vi "subkruispuntbocht.vi"(10 "control 123":i32, 11 "lijn gedetecteerd":bool) -> (9 "einde keuze":bool)   [LabVIEW 2019]
uses:
  <vilib>/myRIO/Common/Instrument Driver Framework/Utilities/typedefs/Analog Scaling Constants.ctl
  <vilib>/myRIO/Common/Instrument Driver Framework/Utilities/typedefs/Analog Scaling Constants List.ctl
  <vilib>/myRIO/Common/Instrument Driver Framework/myRIO v1.0/AO/typedefs/AO Channels Enum.ctl
  <vilib>/myRIO/Common/Instrument Driver Framework/myRIO v1.0/AO/typedefs/AO Channels List.ctl
  <vilib>/myRIO/Common/Instrument Driver Framework/Utilities/typedefs/Generic FPGA Reference.ctl
  <vilib>/myRIO/Common/Instrument Driver Framework/Utilities/typedefs/myRIO v1.0 Reference.ctl
  <vilib>/myRIO/Common/Instrument Driver Framework/Utilities/typedefs/Hardware Version Enum.ctl
  <vilib>/myRIO/Common/Instrument Driver Framework/Utilities/typedefs/myRIO Generic Hardware Reference.ctl
  <vilib>/myRIO/Instrument Drivers/Onboard IO/AO/typedefs/AO Reference.ctl
  <vilib>/myRIO/Instrument Drivers/Onboard IO/AO/AO.lvlib
  <vilib>/myRIO/Instrument Drivers/Onboard IO/AO/vis/Write.vi
  <vilib>/userDefined/High Color/nirio_resource_hc.ctl
  <vilib>/myRIO/Common/Instrument Driver Framework/myRIO v1.0/AO/vis/myRIO v1.1 Open AO.vi
  <vilib>/myRIO/Instrument Drivers/Onboard IO/AO/vis/myRIO AO Open.xnode
  <vilib>/myRIO/Common/Instrument Driver Framework/Utilities/vis/Is FPGA Ref Available.vi
  <vilib>/myRIO/Express VI/Onboard IO/AO/AO Express VI.xnode
  <vilib>/myRIO/Common/Instrument Driver Framework/myRIO v1.0/DIO/typedefs/DIO Channels Enum.ctl
  <vilib>/myRIO/Common/Instrument Driver Framework/myRIO v1.0/DIO/typedefs/DIO Channels List.ctl
  <vilib>/myRIO/Instrument Drivers/Onboard IO/DIO/typedefs/DIO Reference.ctl
  <vilib>/myRIO/Instrument Drivers/Onboard IO/DIO/DIO.lvlib
  <vilib>/myRIO/Instrument Drivers/Onboard IO/DIO/vis/Read.vi
  <vilib>/myRIO/Common/Instrument Driver Framework/myRIO v1.0/DIO/vis/myRIO v1.1 Open DIO.vi
  <vilib>/myRIO/Instrument Drivers/Onboard IO/DIO/vis/myRIO DIO Open.xnode
  <vilib>/myRIO/Express VI/Onboard IO/DI/DI Express VI.xnode
  <vilib>/myRIO/Instrument Drivers/Onboard IO/I2C/typedefs/I2C Transfer Rate.ctl
  <vilib>/myRIO/Instrument Drivers/Onboard IO/I2C/I2C.lvlib
  <vilib>/myRIO/Instrument Drivers/Onboard IO/I2C/typedefs/I2C User Configuration.ctl
  <vilib>/myRIO/Instrument Drivers/Onboard IO/I2C/typedefs/I2C Configuration.ctl
  <vilib>/myRIO/Common/Instrument Driver Framework/myRIO v1.0/I2C/typedefs/I2C Channels Enum.ctl
  <vilib>/myRIO/Instrument Drivers/Onboard IO/I2C/typedefs/I2C Reference.ctl
  <vilib>/myRIO/Instrument Drivers/Onboard IO/I2C/vis/Configure.vi
  <vilib>/myRIO/Instrument Drivers/Onboard IO/I2C/vis/Write.vi
  <vilib>/myRIO/Common/Instrument Driver Framework/myRIO v1.0/I2C/vis/myRIO v1.1 Open I2C.vi
  <vilib>/myRIO/Instrument Drivers/Onboard IO/I2C/vis/myRIO I2C Open.xnode
  <vilib>/myRIO/Express VI/Onboard IO/I2C/I2C Express VI.xnode
  stopkruispunt.vi
panel:
  out "rood  5":u32
  out "rood  4":u32
  out "rood  3":u32
  in  "error in (no error) 4":errorcluster
  out "error out 4":errorcluster
  in  "error in (no error) 3":errorcluster
  out "error out 3":errorcluster
  in  "error in (no error) 2":errorcluster
  out "error out 2":errorcluster
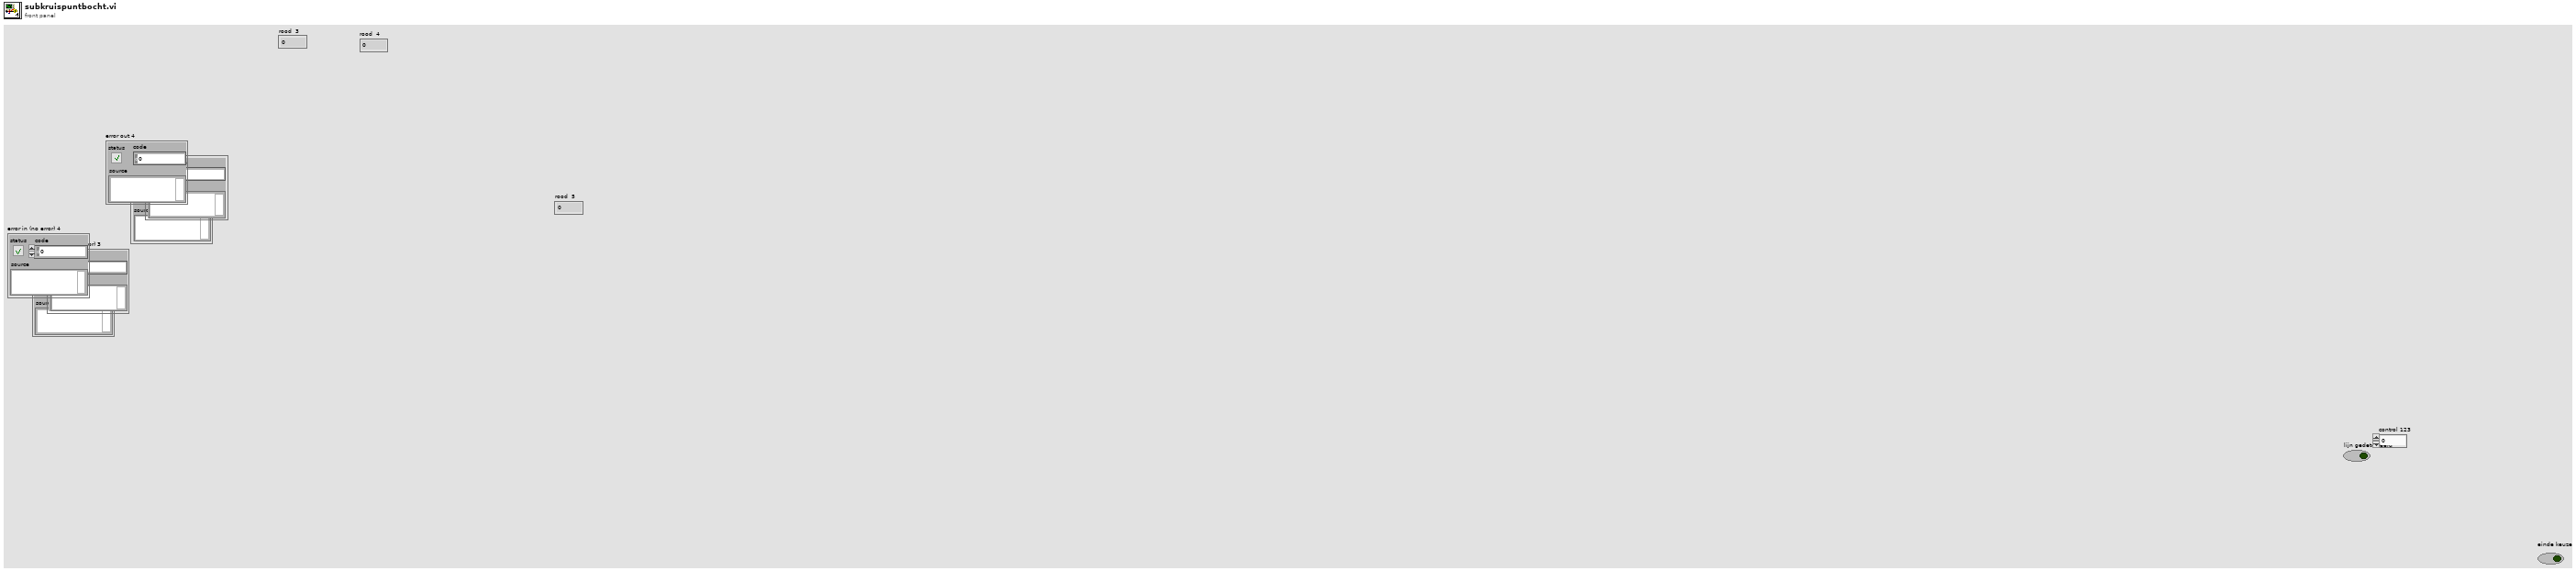
[diagram p1: front panel]
types:
  T1 = typedef "AO.lvlib/AO Reference.ctl" = cluster{"myRIO Reference":T2, "AO Channel List":T6, "AO Scaling Constant List":T8}
  T2 = typedef "myRIO Generic Hardware Reference.ctl" = cluster{"myRIO Model":T3, "myRIO Hardware Reference":T4}
  T3 = typedef "Hardware Version Enum.ctl" = enum16{"Unknown", "myRIO-1900", "myRIO-1950", "roboRIO", "NI ELVIS RIO CM", "ELVIS III"}
  T4 = typedef "myRIO v1.0 Reference.ctl" = cluster{"Generic FPGA Reference":T5, "Allow multiple opens":bool}
  T5 = typedef "Generic FPGA Reference.ctl" = refnum<k20>
  T6 = typedef "AO Channels List.ctl" = T7[]
  T7 = typedef "AO Channels Enum.ctl" = enum16{"Not Connected", "AudioOut/Left", "AudioOut/Right", "C/AO0", "C/AO1", "A/AO0", "A/AO1", "B/AO0", "B/AO1"}
  T8 = typedef "Analog Scaling Constants List.ctl" = T9[]
  T9 = typedef "Analog Scaling Constants.ctl" = cluster{"LSB Weight (Volts)":dbl, "Offset (Volts)":dbl, "Signed?":bool}
  T10 = typedef "nirio_resource_hc.ctl" = tag
  T11 = typedef "I2C.lvlib/I2C Reference.ctl" = cluster{"myRIO Reference":T2, "I2C Channels Enum":T12, "I2C Configuration":T13}
  T12 = typedef "I2C Channels Enum.ctl" = enum16{"Not Connected", "A/I2C", "B/I2C", "I2C/I2C"}
  T13 = typedef "I2C.lvlib/I2C Configuration.ctl" = cluster{"I2C Transfer Rate":T14}
  T14 = typedef "I2C.lvlib/I2C Transfer Rate.ctl" = enum16{"Standard mode (100 kbps)", "Fast mode (400 kbps)"}
  T15 = typedef "I2C.lvlib/I2C User Configuration.ctl" = cluster{"I2C Transfer Rate":T14}
  T16 = typedef "DIO.lvlib/DIO Reference.ctl" = cluster{"myRIO Reference":T2, "DIO Channels List":T17}
  T17 = typedef "DIO Channels List.ctl" = T18[]
  T18 = typedef "DIO Channels Enum.ctl" = enum16{"Not Connected", "C/DIO0", "C/DIO1", "C/DIO2", "C/DIO3", "C/DIO4", "C/DIO5", "C/DIO6", "C/DIO7", "A/DIO0", "A/DIO1", "A/DIO2", "A/DIO3", "A/DIO4", "A/DIO5", "A/DIO6", "A/DIO7", "A/DIO8", "A/DIO9", "A/DIO10", "A/DIO11", "A/DIO12", "A/DIO13", "A/DIO14", "A/DIO15", "A/DIO16", "A/DIO17", "A/DIO18", "A/DIO19", "B/DIO0", "B/DIO1", "B/DIO2", "B/DIO3", "B/DIO4", "B/DIO5", "B/DIO6", "B/DIO7", "B/DIO8", "B/DIO9", "B/DIO10", "B/DIO11", "B/DIO12", "B/DIO13", "B/DIO14", "B/DIO15", "B/DIO16", "B/DIO17", "B/DIO18", "B/DIO19", "LED0", "LED1", "LED2", "LED3", "Button0", "DIO/DIO0", "DIO/DIO1", "DIO/DIO2", "DIO/DIO3", "DIO/DIO4", "DIO/DIO5", "DIO/DIO6", "DIO/DIO7", "DIO/DIO8", "DIO/DIO9", "SPI/CS0", "SPI/CS1", "SPI/CS2", "SPI/CS3", "LED RADIO (Green)", "LED RADIO (Red)", "LED COMM (Green)", "LED COMM (Red)", "LED MODE (Green)", "LED MODE (Red)"}
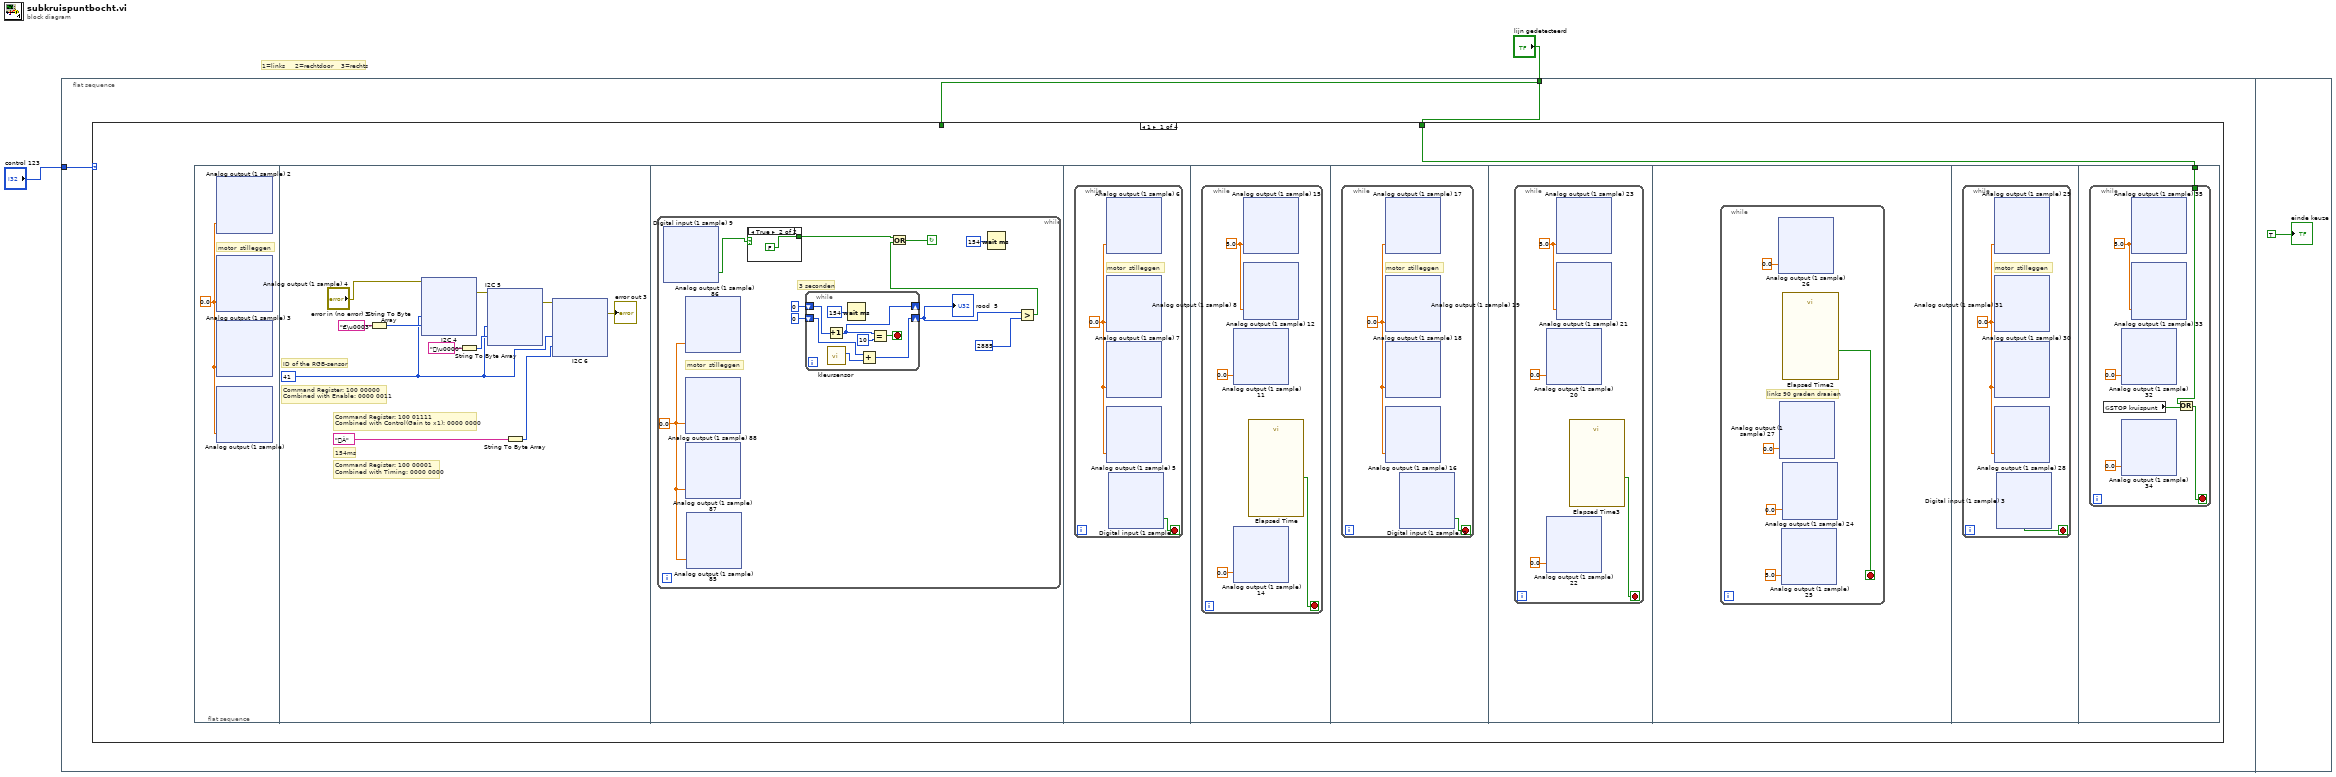
[diagram p0: block diagram]
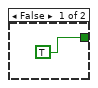
[diagram p2: hidden frame]
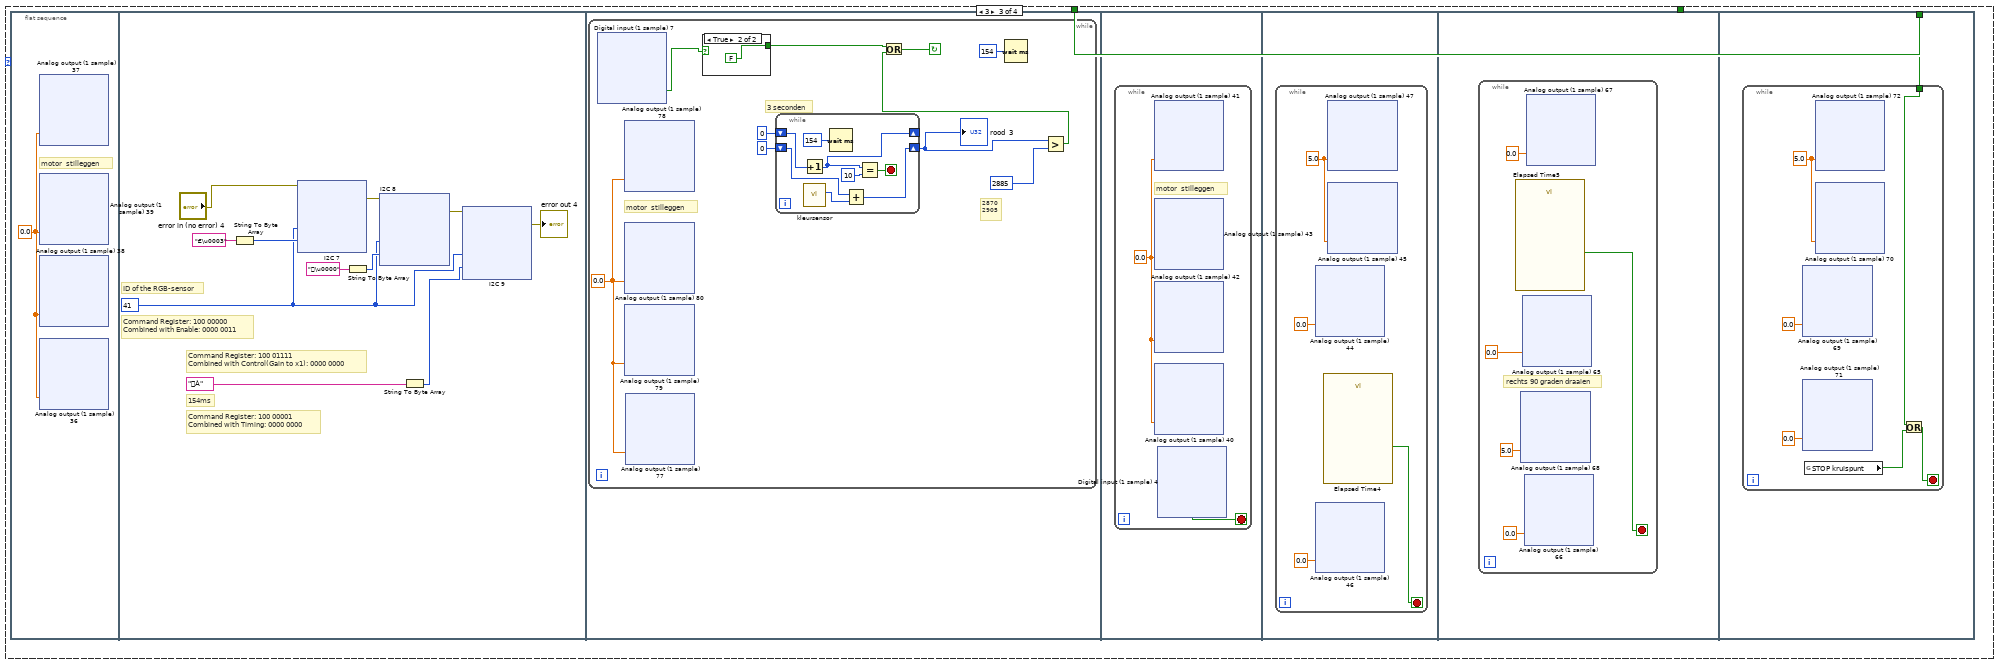
[diagram p4: hidden frame]
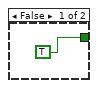
[diagram p5: hidden frame]
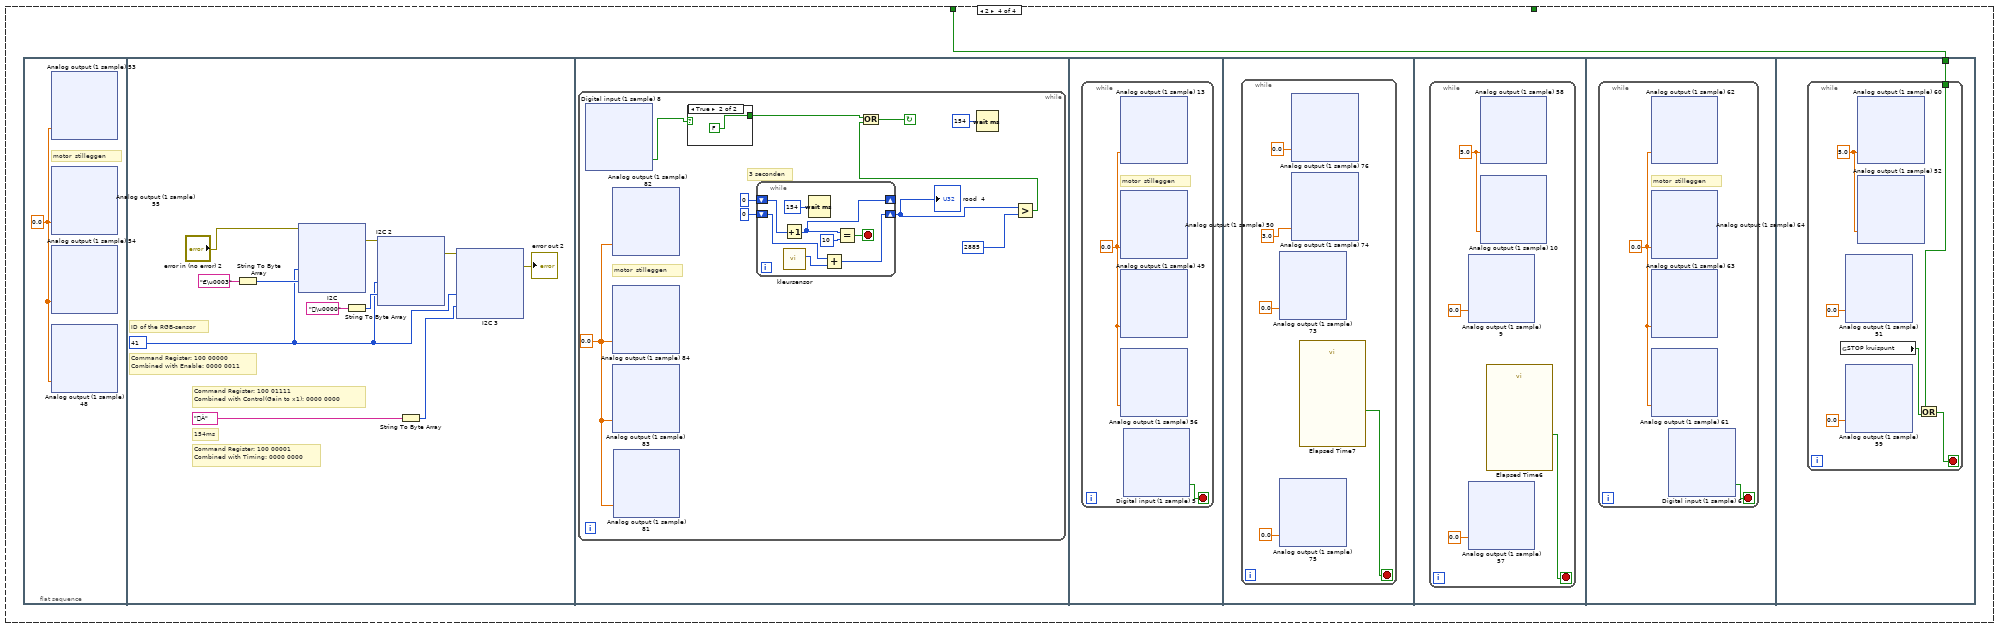
[diagram p6: hidden frame]
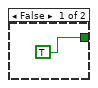
[diagram p7: hidden frame]
diagram:
  # "1=links     2=rechtdoor    3=rechts"
  n1 = flat-sequence {
    tunnel: "lijn gedetecteerd" -> [w4]
    tunnel: "control 123" -> [w3]
    frame #0 {
      n2 = case shown="1" w3 {
        tunnel: w4 -> [w5 _ _ _]
        tunnel: w4 -> [_ _ w1650 w2773]
        frame 1 {
          n3 = flat-sequence {
            tunnel: w5 -> [w1495]
            frame #0 {
              w6 = 0.0
              # "motor  stilleggen"
              n4 = xnode "Analog output (1 sample) 2"("A/AO1 (Pin 4)"=w6) -> ()  [unwired: 1 in, 1 out]
              n5 = xnode "Analog output (1 sample) 4"("B/AO0 (Pin 2)"=w6) -> ()  [unwired: 1 in, 1 out]
              n6 = xnode "Analog output (1 sample) 3"("A/AO0 (Pin 2)"=w6) -> ()  [unwired: 1 in, 1 out]
              n7 = xnode "Analog output (1 sample)"("B/AO1 (Pin 4)"=w6) -> ()  [unwired: 1 in, 1 out]
            }
            frame #1 {
              w158 = 41 ("Numeric")
              # "154ms"
              # "ID of the RGB-sensor"
              # "Command Register: 100 00000\nCombined with Enable: 0000 0011"
              # "Command Register: 100 01111\nCombined with Control(Gain to x1): 0000 0000"
              # "Command Register: 100 00001\nCombined with Timing: 0000 0000"
              n8 = String To Byte Array(string="€\u0003") -> (unsigned byte array=w165:u8[])
              n9 = xnode "I2C 4"("Slave Address (7-bit)"=w158, "Bytes to Write"=w165, "error in (no error)"="error in (no error) 3") -> ("error out"=w162:errorcluster)
              n10 = String To Byte Array(string="\u0000") -> (unsigned byte array=w164:u8[])
              n11 = xnode "I2C 5"("Slave Address (7-bit)"=w158, "Bytes to Write"=w164, "error in (no error)"=w162) -> ("error out"=w161:errorcluster)
              n12 = String To Byte Array(string="À") -> (unsigned byte array=w163:u8[])
              n13 = xnode "I2C 6"("Slave Address (7-bit)"=w158, "Bytes to Write"=w163, "error in (no error)"=w161) -> ("error out"=→"error out 3":errorcluster)
            }
            frame #2 {
              n14 = while {
                stop <- w285 continue-if-true
                w289 = 0.0
                # "3 seconden"
                # "motor  stilleggen"
                n15 = xnode "Digital input (1 sample) 9"() -> ("A/DIO1 (Pin 13)"=w283:bool)  [unwired: 1 in, 1 out]
                n16 = xnode "Analog output (1 sample) 86"("A/AO1 (Pin 4)"=w289) -> ()  [unwired: 1 in, 1 out]
                n17 = xnode "Analog output (1 sample) 88"("B/AO0 (Pin 2)"=w289) -> ()  [unwired: 1 in, 1 out]
                n18 = xnode "Analog output (1 sample) 87"("A/AO0 (Pin 2)"=w289) -> ()  [unwired: 1 in, 1 out]
                n19 = xnode "Analog output (1 sample) 85"("B/AO1 (Pin 4)"=w289) -> ()  [unwired: 1 in, 1 out]
                n20 = case shown="True" w283 {
                  tunnel: [TRUE FALSE] -> w282
                  frame False {
                  }
                  frame True {
                  }
                }
                n21 = while {
                  shift-right: [w296] -> _
                  shift-left: 0 -> [w298]
                  shift-right: [w292] -> w288
                  shift-left: 0 -> [w294]
                  stop <- w297 stop-if-true
                  n22 = Increment(x=w298) -> (x+1=w296:i32)
                  n23 = call "kleursensor.vi"() -> ("Total 2"=w293:u32)  [unwired: 8 in, 3 out]
                  n24 = Wait (ms)(milliseconds to wait=u32 154) -> ()  [unwired: 1 out]
                  n25 = Add(x=w294, y=w293) -> (x+y=w292:u32)
                  n26 = Equal?(x=w296, y=10) -> (x = y?=w297:bool)
                }
                "rood  5" <- w288
                n27 = Wait (ms)(milliseconds to wait=u32 154) -> ()  [unwired: 1 out]
                n28 = Greater?(x=w288, y=2885) -> (0:w284:bool)
                n29 = Or(x=w282, y=w284) -> (x .or. y?=w285:bool)
              }
            }
            frame #3 {
              n30 = while {
                stop <- w483 stop-if-true
                w484 = 0.0
                # "motor  stilleggen"
                n31 = xnode "Analog output (1 sample) 6"("A/AO1 (Pin 4)"=w484) -> ()  [unwired: 1 in, 1 out]
                n32 = xnode "Analog output (1 sample) 8"("B/AO0 (Pin 2)"=w484) -> ()  [unwired: 1 in, 1 out]
                n33 = xnode "Analog output (1 sample) 7"("A/AO0 (Pin 2)"=w484) -> ()  [unwired: 1 in, 1 out]
                n34 = xnode "Analog output (1 sample) 5"("B/AO1 (Pin 4)"=w484) -> ()  [unwired: 1 in, 1 out]
                n35 = xnode "Digital input (1 sample)"() -> ("A/DIO1 (Pin 13)"=w483:bool)  [unwired: 1 in, 1 out]
              }
            }
            frame #4 {
              n36 = while {
                stop <- w668 stop-if-true
                w670 = 5.0
                n37 = xnode "Analog output (1 sample) 11"("B/AO1 (Pin 4)"=0.0) -> ()  [unwired: 1 in, 1 out]
                n38 = xnode "Analog output (1 sample) 14"("A/AO1 (Pin 4)"=0.0) -> ()  [unwired: 1 in, 1 out]
                n39 = xnode "Analog output (1 sample) 15"("A/AO0 (Pin 2)"=w670) -> ()  [unwired: 1 in, 1 out]
                n40 = xnode "Analog output (1 sample) 12"("B/AO0 (Pin 2)"=w670) -> ()  [unwired: 1 in, 1 out]
                n41 = call "Elapsed Time"() -> ("Time has Elapsed"=w668:bool)  [unwired: 12 in, 7 out]
              }
            }
            frame #5 {
              n42 = while {
                stop <- w821 stop-if-true
                w820 = 0.0
                # "motor  stilleggen"
                n43 = xnode "Analog output (1 sample) 17"("A/AO1 (Pin 4)"=w820) -> ()  [unwired: 1 in, 1 out]
                n44 = xnode "Analog output (1 sample) 19"("B/AO0 (Pin 2)"=w820) -> ()  [unwired: 1 in, 1 out]
                n45 = xnode "Analog output (1 sample) 18"("A/AO0 (Pin 2)"=w820) -> ()  [unwired: 1 in, 1 out]
                n46 = xnode "Analog output (1 sample) 16"("B/AO1 (Pin 4)"=w820) -> ()  [unwired: 1 in, 1 out]
                n47 = xnode "Digital input (1 sample) 2"() -> ("A/DIO1 (Pin 13)"=w821:bool)  [unwired: 1 in, 1 out]
              }
            }
            frame #6 {
              n48 = while {
                stop <- w1005 stop-if-true
                w1007 = 5.0
                n49 = xnode "Analog output (1 sample) 20"("B/AO1 (Pin 4)"=0.0) -> ()  [unwired: 1 in, 1 out]
                n50 = xnode "Analog output (1 sample) 22"("A/AO1 (Pin 4)"=0.0) -> ()  [unwired: 1 in, 1 out]
                n51 = xnode "Analog output (1 sample) 23"("A/AO0 (Pin 2)"=w1007) -> ()  [unwired: 1 in, 1 out]
                n52 = xnode "Analog output (1 sample) 21"("B/AO0 (Pin 2)"=w1007) -> ()  [unwired: 1 in, 1 out]
                n53 = call "Elapsed Time3"() -> ("Time has Elapsed"=w1005:bool)  [unwired: 12 in, 7 out]
              }
            }
            frame #7 {
              n54 = while {
                stop <- w1157 stop-if-true
                # "links 90 graden draaien"
                n55 = xnode "Analog output (1 sample) 26"("A/AO1 (Pin 4)"=0.0) -> ()  [unwired: 1 in, 1 out]
                n56 = xnode "Analog output (1 sample) 27"("A/AO0 (Pin 2)"=0.0) -> ()  [unwired: 1 in, 1 out]
                n57 = xnode "Analog output (1 sample) 25"("B/AO0 (Pin 2)"=5.0) -> ()  [unwired: 1 in, 1 out]
                n58 = xnode "Analog output (1 sample) 24"("B/AO1 (Pin 4)"=0.0) -> ()  [unwired: 1 in, 1 out]
                n59 = call "Elapsed Time2"() -> ("Time has Elapsed"=w1157:bool)  [unwired: 12 in, 7 out]
              }
            }
            frame #8 {
              n60 = while {
                stop <- w1311 stop-if-true
                w1310 = 0.0
                # "motor  stilleggen"
                n61 = xnode "Analog output (1 sample) 29"("A/AO1 (Pin 4)"=w1310) -> ()  [unwired: 1 in, 1 out]
                n62 = xnode "Analog output (1 sample) 31"("B/AO0 (Pin 2)"=w1310) -> ()  [unwired: 1 in, 1 out]
                n63 = xnode "Analog output (1 sample) 30"("A/AO0 (Pin 2)"=w1310) -> ()  [unwired: 1 in, 1 out]
                n64 = xnode "Analog output (1 sample) 28"("B/AO1 (Pin 4)"=w1310) -> ()  [unwired: 1 in, 1 out]
                n65 = xnode "Digital input (1 sample) 3"() -> ("A/DIO1 (Pin 13)"=w1311:bool)  [unwired: 1 in, 1 out]
              }
            }
            frame #9 {
              n66 = while {
                tunnel: w1495 -> [w1497]
                stop <- w1496 stop-if-true
                w1500 = 5.0
                n67 = global read "stopkruispunt.vi" "STOP kruispunt"() -> (w1498:bool)
                n68 = xnode "Analog output (1 sample) 32"("B/AO1 (Pin 4)"=0.0) -> ()  [unwired: 1 in, 1 out]
                n69 = xnode "Analog output (1 sample) 34"("A/AO1 (Pin 4)"=0.0) -> ()  [unwired: 1 in, 1 out]
                n70 = xnode "Analog output (1 sample) 35"("A/AO0 (Pin 2)"=w1500) -> ()  [unwired: 1 in, 1 out]
                n71 = xnode "Analog output (1 sample) 33"("B/AO0 (Pin 2)"=w1500) -> ()  [unwired: 1 in, 1 out]
                n72 = Or(x=w1497, y=w1498) -> (x .or. y?=w1496:bool)
              }
            }
          }
        }
        frame 4, Default {
        }
        frame 3 {
          n73 = flat-sequence {
            tunnel: w1650 -> [w2618]
            frame #0 {
              w1651 = 0.0
              # "motor  stilleggen"
              n74 = xnode "Analog output (1 sample) 37"("A/AO1 (Pin 4)"=w1651) -> ()  [unwired: 1 in, 1 out]
              n75 = xnode "Analog output (1 sample) 39"("B/AO0 (Pin 2)"=w1651) -> ()  [unwired: 1 in, 1 out]
              n76 = xnode "Analog output (1 sample) 38"("A/AO0 (Pin 2)"=w1651) -> ()  [unwired: 1 in, 1 out]
              n77 = xnode "Analog output (1 sample) 36"("B/AO1 (Pin 4)"=w1651) -> ()  [unwired: 1 in, 1 out]
            }
            frame #1 {
              w1803 = 41 ("Numeric")
              # "154ms"
              # "ID of the RGB-sensor"
              # "Command Register: 100 00000\nCombined with Enable: 0000 0011"
              # "Command Register: 100 01111\nCombined with Control(Gain to x1): 0000 0000"
              # "Command Register: 100 00001\nCombined with Timing: 0000 0000"
              n78 = String To Byte Array(string="€\u0003") -> (unsigned byte array=w1810:u8[])
              n79 = xnode "I2C 7"("Slave Address (7-bit)"=w1803, "Bytes to Write"=w1810, "error in (no error)"="error in (no error) 4") -> ("error out"=w1807:errorcluster)
              n80 = String To Byte Array(string="\u0000") -> (unsigned byte array=w1809:u8[])
              n81 = xnode "I2C 8"("Slave Address (7-bit)"=w1803, "Bytes to Write"=w1809, "error in (no error)"=w1807) -> ("error out"=w1806:errorcluster)
              n82 = String To Byte Array(string="À") -> (unsigned byte array=w1808:u8[])
              n83 = xnode "I2C 9"("Slave Address (7-bit)"=w1803, "Bytes to Write"=w1808, "error in (no error)"=w1806) -> ("error out"=→"error out 4":errorcluster)
            }
            frame #2 {
              n84 = while {
                stop <- w1930 continue-if-true
                w1934 = 0.0
                # "2870\n2905"
                # "3 seconden"
                # "motor  stilleggen"
                n85 = xnode "Digital input (1 sample) 7"() -> ("A/DIO1 (Pin 13)"=w1928:bool)  [unwired: 1 in, 1 out]
                n86 = xnode "Analog output (1 sample) 78"("A/AO1 (Pin 4)"=w1934) -> ()  [unwired: 1 in, 1 out]
                n87 = xnode "Analog output (1 sample) 80"("B/AO0 (Pin 2)"=w1934) -> ()  [unwired: 1 in, 1 out]
                n88 = xnode "Analog output (1 sample) 79"("A/AO0 (Pin 2)"=w1934) -> ()  [unwired: 1 in, 1 out]
                n89 = xnode "Analog output (1 sample) 77"("B/AO1 (Pin 4)"=w1934) -> ()  [unwired: 1 in, 1 out]
                n90 = case shown="True" w1928 {
                  tunnel: [TRUE FALSE] -> w1927
                  frame False {
                  }
                  frame True {
                  }
                }
                n91 = while {
                  shift-right: [w1941] -> _
                  shift-left: 0 -> [w1943]
                  shift-right: [w1937] -> w1933
                  shift-left: 0 -> [w1939]
                  stop <- w1942 stop-if-true
                  n92 = Increment(x=w1943) -> (x+1=w1941:i32)
                  n93 = call "kleursensor.vi"() -> ("Total 2"=w1938:u32)  [unwired: 8 in, 3 out]
                  n94 = Wait (ms)(milliseconds to wait=u32 154) -> ()  [unwired: 1 out]
                  n95 = Add(x=w1939, y=w1938) -> (x+y=w1937:u32)
                  n96 = Equal?(x=w1941, y=10) -> (x = y?=w1942:bool)
                }
                "rood  3" <- w1933
                n97 = Wait (ms)(milliseconds to wait=u32 154) -> ()  [unwired: 1 out]
                n98 = Greater?(x=w1933, y=2885) -> (0:w1929:bool)
                n99 = Or(x=w1927, y=w1929) -> (x .or. y?=w1930:bool)
              }
            }
            frame #3 {
              n100 = while {
                stop <- w2128 stop-if-true
                w2129 = 0.0
                # "motor  stilleggen"
                n101 = xnode "Analog output (1 sample) 41"("A/AO1 (Pin 4)"=w2129) -> ()  [unwired: 1 in, 1 out]
                n102 = xnode "Analog output (1 sample) 43"("B/AO0 (Pin 2)"=w2129) -> ()  [unwired: 1 in, 1 out]
                n103 = xnode "Analog output (1 sample) 42"("A/AO0 (Pin 2)"=w2129) -> ()  [unwired: 1 in, 1 out]
                n104 = xnode "Analog output (1 sample) 40"("B/AO1 (Pin 4)"=w2129) -> ()  [unwired: 1 in, 1 out]
                n105 = xnode "Digital input (1 sample) 4"() -> ("A/DIO1 (Pin 13)"=w2128:bool)  [unwired: 1 in, 1 out]
              }
            }
            frame #4 {
              n106 = while {
                stop <- w2313 stop-if-true
                w2315 = 5.0
                n107 = xnode "Analog output (1 sample) 44"("B/AO1 (Pin 4)"=0.0) -> ()  [unwired: 1 in, 1 out]
                n108 = xnode "Analog output (1 sample) 46"("A/AO1 (Pin 4)"=0.0) -> ()  [unwired: 1 in, 1 out]
                n109 = call "Elapsed Time4"() -> ("Time has Elapsed"=w2313:bool)  [unwired: 12 in, 7 out]
                n110 = xnode "Analog output (1 sample) 47"("A/AO0 (Pin 2)"=w2315) -> ()  [unwired: 1 in, 1 out]
                n111 = xnode "Analog output (1 sample) 45"("B/AO0 (Pin 2)"=w2315) -> ()  [unwired: 1 in, 1 out]
              }
            }
            frame #5 {
              n112 = while {
                stop <- w2465 stop-if-true
                # "rechts 90 graden draaien"
                n113 = call "Elapsed Time5"() -> ("Time has Elapsed"=w2465:bool)  [unwired: 12 in, 7 out]
                n114 = xnode "Analog output (1 sample) 68"("A/AO0 (Pin 2)"=5.0) -> ()  [unwired: 1 in, 1 out]
                n115 = xnode "Analog output (1 sample) 65"("B/AO1 (Pin 4)"=0.0) -> ()  [unwired: 1 in, 1 out]
                n116 = xnode "Analog output (1 sample) 66"("B/AO0 (Pin 2)"=0.0) -> ()  [unwired: 1 in, 1 out]
                n117 = xnode "Analog output (1 sample) 67"("A/AO1 (Pin 4)"=0.0) -> ()  [unwired: 1 in, 1 out]
              }
            }
            frame #6 {
              n118 = while {
                tunnel: w2618 -> [w2620]
                stop <- w2621 stop-if-true
                w2623 = 5.0
                n119 = xnode "Analog output (1 sample) 69"("B/AO1 (Pin 4)"=0.0) -> ()  [unwired: 1 in, 1 out]
                n120 = xnode "Analog output (1 sample) 71"("A/AO1 (Pin 4)"=0.0) -> ()  [unwired: 1 in, 1 out]
                n121 = global read "stopkruispunt.vi" "STOP kruispunt"() -> (w2619:bool)
                n122 = xnode "Analog output (1 sample) 72"("A/AO0 (Pin 2)"=w2623) -> ()  [unwired: 1 in, 1 out]
                n123 = xnode "Analog output (1 sample) 70"("B/AO0 (Pin 2)"=w2623) -> ()  [unwired: 1 in, 1 out]
                n124 = Or(x=w2620, y=w2619) -> (x .or. y?=w2621:bool)
              }
            }
          }
        }
        frame 2 {
          n125 = flat-sequence {
            tunnel: w2773 -> [w3926]
            frame #0 {
              w2774 = 0.0
              # "motor  stilleggen"
              n126 = xnode "Analog output (1 sample) 53"("A/AO1 (Pin 4)"=w2774) -> ()  [unwired: 1 in, 1 out]
              n127 = xnode "Analog output (1 sample) 55"("B/AO0 (Pin 2)"=w2774) -> ()  [unwired: 1 in, 1 out]
              n128 = xnode "Analog output (1 sample) 54"("A/AO0 (Pin 2)"=w2774) -> ()  [unwired: 1 in, 1 out]
              n129 = xnode "Analog output (1 sample) 48"("B/AO1 (Pin 4)"=w2774) -> ()  [unwired: 1 in, 1 out]
            }
            frame #1 {
              w2926 = 41 ("Numeric")
              # "154ms"
              # "ID of the RGB-sensor"
              # "Command Register: 100 00000\nCombined with Enable: 0000 0011"
              # "Command Register: 100 01111\nCombined with Control(Gain to x1): 0000 0000"
              # "Command Register: 100 00001\nCombined with Timing: 0000 0000"
              n130 = String To Byte Array(string="€\u0003") -> (unsigned byte array=w2933:u8[])
              n131 = xnode "I2C"("Slave Address (7-bit)"=w2926, "Bytes to Write"=w2933, "error in (no error)"="error in (no error) 2") -> ("error out"=w2930:errorcluster)
              n132 = String To Byte Array(string="\u0000") -> (unsigned byte array=w2932:u8[])
              n133 = xnode "I2C 2"("Slave Address (7-bit)"=w2926, "Bytes to Write"=w2932, "error in (no error)"=w2930) -> ("error out"=w2929:errorcluster)
              n134 = String To Byte Array(string="À") -> (unsigned byte array=w2931:u8[])
              n135 = xnode "I2C 3"("Slave Address (7-bit)"=w2926, "Bytes to Write"=w2931, "error in (no error)"=w2929) -> ("error out"=→"error out 2":errorcluster)
            }
            frame #2 {
              n136 = while {
                stop <- w3053 continue-if-true
                w3057 = 0.0
                # "3 seconden"
                # "motor  stilleggen"
                n137 = xnode "Digital input (1 sample) 8"() -> ("A/DIO1 (Pin 13)"=w3051:bool)  [unwired: 1 in, 1 out]
                n138 = xnode "Analog output (1 sample) 82"("A/AO1 (Pin 4)"=w3057) -> ()  [unwired: 1 in, 1 out]
                n139 = xnode "Analog output (1 sample) 84"("B/AO0 (Pin 2)"=w3057) -> ()  [unwired: 1 in, 1 out]
                n140 = xnode "Analog output (1 sample) 83"("A/AO0 (Pin 2)"=w3057) -> ()  [unwired: 1 in, 1 out]
                n141 = xnode "Analog output (1 sample) 81"("B/AO1 (Pin 4)"=w3057) -> ()  [unwired: 1 in, 1 out]
                n142 = case shown="True" w3051 {
                  tunnel: [TRUE FALSE] -> w3050
                  frame False {
                  }
                  frame True {
                  }
                }
                n143 = while {
                  shift-right: [w3064] -> _
                  shift-left: 0 -> [w3066]
                  shift-right: [w3060] -> w3056
                  shift-left: 0 -> [w3062]
                  stop <- w3065 stop-if-true
                  n144 = Increment(x=w3066) -> (x+1=w3064:i32)
                  n145 = call "kleursensor.vi"() -> ("Total 2"=w3061:u32)  [unwired: 8 in, 3 out]
                  n146 = Wait (ms)(milliseconds to wait=u32 154) -> ()  [unwired: 1 out]
                  n147 = Add(x=w3062, y=w3061) -> (x+y=w3060:u32)
                  n148 = Equal?(x=w3064, y=10) -> (x = y?=w3065:bool)
                }
                "rood  4" <- w3056
                n149 = Wait (ms)(milliseconds to wait=u32 154) -> ()  [unwired: 1 out]
                n150 = Greater?(x=w3056, y=2885) -> (0:w3052:bool)
                n151 = Or(x=w3050, y=w3052) -> (x .or. y?=w3053:bool)
              }
            }
            frame #3 {
              n152 = while {
                stop <- w3251 stop-if-true
                w3252 = 0.0
                # "motor  stilleggen"
                n153 = xnode "Analog output (1 sample) 13"("A/AO1 (Pin 4)"=w3252) -> ()  [unwired: 1 in, 1 out]
                n154 = xnode "Analog output (1 sample) 50"("B/AO0 (Pin 2)"=w3252) -> ()  [unwired: 1 in, 1 out]
                n155 = xnode "Analog output (1 sample) 49"("A/AO0 (Pin 2)"=w3252) -> ()  [unwired: 1 in, 1 out]
                n156 = xnode "Analog output (1 sample) 56"("B/AO1 (Pin 4)"=w3252) -> ()  [unwired: 1 in, 1 out]
                n157 = xnode "Digital input (1 sample) 5"() -> ("A/DIO1 (Pin 13)"=w3251:bool)  [unwired: 1 in, 1 out]
              }
            }
            frame #4 {
              n158 = while {
                stop <- w3437 stop-if-true
                n159 = xnode "Analog output (1 sample) 73"("B/AO1 (Pin 4)"=0.0) -> ()  [unwired: 1 in, 1 out]
                n160 = xnode "Analog output (1 sample) 75"("A/AO1 (Pin 4)"=0.0) -> ()  [unwired: 1 in, 1 out]
                n161 = xnode "Analog output (1 sample) 76"("A/AO0 (Pin 2)"=0.0) -> ()  [unwired: 1 in, 1 out]
                n162 = xnode "Analog output (1 sample) 74"("B/AO0 (Pin 2)"=3.0) -> ()  [unwired: 1 in, 1 out]
                n163 = call "Elapsed Time7"() -> ("Time has Elapsed"=w3437:bool)  [unwired: 12 in, 7 out]
              }
            }
            frame #5 {
              n164 = while {
                stop <- w3589 stop-if-true
                w3591 = 5.0
                n165 = xnode "Analog output (1 sample) 9"("B/AO1 (Pin 4)"=0.0) -> ()  [unwired: 1 in, 1 out]
                n166 = xnode "Analog output (1 sample) 57"("A/AO1 (Pin 4)"=0.0) -> ()  [unwired: 1 in, 1 out]
                n167 = xnode "Analog output (1 sample) 58"("A/AO0 (Pin 2)"=w3591) -> ()  [unwired: 1 in, 1 out]
                n168 = xnode "Analog output (1 sample) 10"("B/AO0 (Pin 2)"=w3591) -> ()  [unwired: 1 in, 1 out]
                n169 = call "Elapsed Time6"() -> ("Time has Elapsed"=w3589:bool)  [unwired: 12 in, 7 out]
              }
            }
            frame #6 {
              n170 = while {
                stop <- w3742 stop-if-true
                w3741 = 0.0
                # "motor  stilleggen"
                n171 = xnode "Analog output (1 sample) 62"("A/AO1 (Pin 4)"=w3741) -> ()  [unwired: 1 in, 1 out]
                n172 = xnode "Analog output (1 sample) 64"("B/AO0 (Pin 2)"=w3741) -> ()  [unwired: 1 in, 1 out]
                n173 = xnode "Analog output (1 sample) 63"("A/AO0 (Pin 2)"=w3741) -> ()  [unwired: 1 in, 1 out]
                n174 = xnode "Analog output (1 sample) 61"("B/AO1 (Pin 4)"=w3741) -> ()  [unwired: 1 in, 1 out]
                n175 = xnode "Digital input (1 sample) 6"() -> ("A/DIO1 (Pin 13)"=w3742:bool)  [unwired: 1 in, 1 out]
              }
            }
            frame #7 {
              n176 = while {
                tunnel: w3926 -> [w3927]
                stop <- w3929 stop-if-true
                w3931 = 5.0
                n177 = global read "stopkruispunt.vi" "STOP kruispunt"() -> (w3928:bool)
                n178 = xnode "Analog output (1 sample) 51"("B/AO1 (Pin 4)"=0.0) -> ()  [unwired: 1 in, 1 out]
                n179 = xnode "Analog output (1 sample) 59"("A/AO1 (Pin 4)"=0.0) -> ()  [unwired: 1 in, 1 out]
                n180 = xnode "Analog output (1 sample) 60"("A/AO0 (Pin 2)"=w3931) -> ()  [unwired: 1 in, 1 out]
                n181 = xnode "Analog output (1 sample) 52"("B/AO0 (Pin 2)"=w3931) -> ()  [unwired: 1 in, 1 out]
                n182 = Or(x=w3927, y=w3928) -> (x .or. y?=w3929:bool)
              }
            }
          }
        }
      }
    }
    frame #1 {
      "einde keuze" <- TRUE
    }
  }
